vi "Draw All Bones.vi"(6 "Color":u32(colorbox)=16711680, 7 "Include Inferred Joints?":bool=TRUE, 8 "error in":errorcluster, 9 "Body Index":i32, 11 "Image":T1) -> (0 "error out":errorcluster, 3 "Image Out":T1)   [LabVIEW 2011, in "LVH-KinectOne.lvlib"]
uses:
  LVH-KinectOne.lvlib
  <vilib>/vision/Image Controls.llb/IMAQ Image.ctl
  Type Defs/JointType.ctl
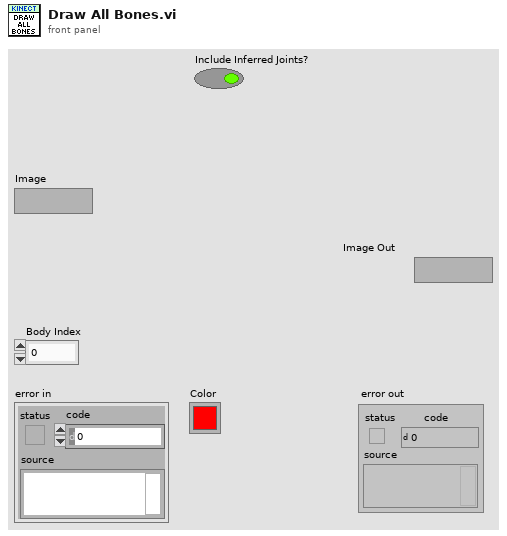
[diagram p1: front panel]
types:
  T1 = typedef "IMAQ Image.ctl" = refnum<image>
  T2 = typedef "LVH-KinectOne.lvlib/JointType.ctl" = i32
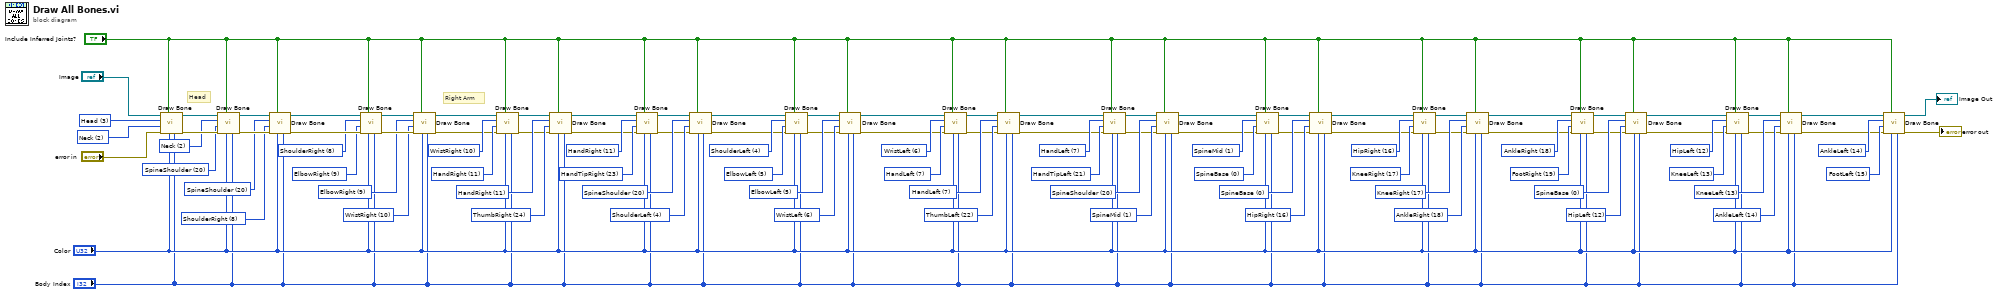
[diagram p0: block diagram]
diagram:
  w9 = T2 15 items=["SpineBase", "SpineMid", "Neck", "Head", "ShoulderLeft", "ElbowLeft", "WristLeft", "HandLeft", "ShoulderRight", "ElbowRight", "WristRight", "HandRight", "HipLeft", "KneeLeft", "AnkleLeft", "FootLeft", "HipRight", "KneeRight", "AnkleRight", "FootRight", "SpineShoulder", "HandTipLeft", "ThumbLeft", "HandTipRight", "ThumbRight"] ("Ending Joint")
  w8 = T2 14 items=["SpineBase", "SpineMid", "Neck", "Head", "ShoulderLeft", "ElbowLeft", "WristLeft", "HandLeft", "ShoulderRight", "ElbowRight", "WristRight", "HandRight", "HipLeft", "KneeLeft", "AnkleLeft", "FootLeft", "HipRight", "KneeRight", "AnkleRight", "FootRight", "SpineShoulder", "HandTipLeft", "ThumbLeft", "HandTipRight", "ThumbRight"] ("Starting Joint")
  w17 = T2 14 items=["SpineBase", "SpineMid", "Neck", "Head", "ShoulderLeft", "ElbowLeft", "WristLeft", "HandLeft", "ShoulderRight", "ElbowRight", "WristRight", "HandRight", "HipLeft", "KneeLeft", "AnkleLeft", "FootLeft", "HipRight", "KneeRight", "AnkleRight", "FootRight", "SpineShoulder", "HandTipLeft", "ThumbLeft", "HandTipRight", "ThumbRight"] ("Ending Joint")
  w16 = T2 13 items=["SpineBase", "SpineMid", "Neck", "Head", "ShoulderLeft", "ElbowLeft", "WristLeft", "HandLeft", "ShoulderRight", "ElbowRight", "WristRight", "HandRight", "HipLeft", "KneeLeft", "AnkleLeft", "FootLeft", "HipRight", "KneeRight", "AnkleRight", "FootRight", "SpineShoulder", "HandTipLeft", "ThumbLeft", "HandTipRight", "ThumbRight"] ("Starting Joint")
  w13 = T2 13 items=["SpineBase", "SpineMid", "Neck", "Head", "ShoulderLeft", "ElbowLeft", "WristLeft", "HandLeft", "ShoulderRight", "ElbowRight", "WristRight", "HandRight", "HipLeft", "KneeLeft", "AnkleLeft", "FootLeft", "HipRight", "KneeRight", "AnkleRight", "FootRight", "SpineShoulder", "HandTipLeft", "ThumbLeft", "HandTipRight", "ThumbRight"] ("Ending Joint")
  w12 = T2 12 items=["SpineBase", "SpineMid", "Neck", "Head", "ShoulderLeft", "ElbowLeft", "WristLeft", "HandLeft", "ShoulderRight", "ElbowRight", "WristRight", "HandRight", "HipLeft", "KneeLeft", "AnkleLeft", "FootLeft", "HipRight", "KneeRight", "AnkleRight", "FootRight", "SpineShoulder", "HandTipLeft", "ThumbLeft", "HandTipRight", "ThumbRight"] ("Starting Joint")
  w25 = T2 12 items=["SpineBase", "SpineMid", "Neck", "Head", "ShoulderLeft", "ElbowLeft", "WristLeft", "HandLeft", "ShoulderRight", "ElbowRight", "WristRight", "HandRight", "HipLeft", "KneeLeft", "AnkleLeft", "FootLeft", "HipRight", "KneeRight", "AnkleRight", "FootRight", "SpineShoulder", "HandTipLeft", "ThumbLeft", "HandTipRight", "ThumbRight"] ("Ending Joint")
  w24 = T2 0 items=["SpineBase", "SpineMid", "Neck", "Head", "ShoulderLeft", "ElbowLeft", "WristLeft", "HandLeft", "ShoulderRight", "ElbowRight", "WristRight", "HandRight", "HipLeft", "KneeLeft", "AnkleLeft", "FootLeft", "HipRight", "KneeRight", "AnkleRight", "FootRight", "SpineShoulder", "HandTipLeft", "ThumbLeft", "HandTipRight", "ThumbRight"] ("Starting Joint")
  w21 = T2 19 items=["SpineBase", "SpineMid", "Neck", "Head", "ShoulderLeft", "ElbowLeft", "WristLeft", "HandLeft", "ShoulderRight", "ElbowRight", "WristRight", "HandRight", "HipLeft", "KneeLeft", "AnkleLeft", "FootLeft", "HipRight", "KneeRight", "AnkleRight", "FootRight", "SpineShoulder", "HandTipLeft", "ThumbLeft", "HandTipRight", "ThumbRight"] ("Ending Joint")
  w20 = T2 18 items=["SpineBase", "SpineMid", "Neck", "Head", "ShoulderLeft", "ElbowLeft", "WristLeft", "HandLeft", "ShoulderRight", "ElbowRight", "WristRight", "HandRight", "HipLeft", "KneeLeft", "AnkleLeft", "FootLeft", "HipRight", "KneeRight", "AnkleRight", "FootRight", "SpineShoulder", "HandTipLeft", "ThumbLeft", "HandTipRight", "ThumbRight"] ("Starting Joint")
  w33 = T2 18 items=["SpineBase", "SpineMid", "Neck", "Head", "ShoulderLeft", "ElbowLeft", "WristLeft", "HandLeft", "ShoulderRight", "ElbowRight", "WristRight", "HandRight", "HipLeft", "KneeLeft", "AnkleLeft", "FootLeft", "HipRight", "KneeRight", "AnkleRight", "FootRight", "SpineShoulder", "HandTipLeft", "ThumbLeft", "HandTipRight", "ThumbRight"] ("Ending Joint")
  w32 = T2 17 items=["SpineBase", "SpineMid", "Neck", "Head", "ShoulderLeft", "ElbowLeft", "WristLeft", "HandLeft", "ShoulderRight", "ElbowRight", "WristRight", "HandRight", "HipLeft", "KneeLeft", "AnkleLeft", "FootLeft", "HipRight", "KneeRight", "AnkleRight", "FootRight", "SpineShoulder", "HandTipLeft", "ThumbLeft", "HandTipRight", "ThumbRight"] ("Starting Joint")
  w29 = T2 17 items=["SpineBase", "SpineMid", "Neck", "Head", "ShoulderLeft", "ElbowLeft", "WristLeft", "HandLeft", "ShoulderRight", "ElbowRight", "WristRight", "HandRight", "HipLeft", "KneeLeft", "AnkleLeft", "FootLeft", "HipRight", "KneeRight", "AnkleRight", "FootRight", "SpineShoulder", "HandTipLeft", "ThumbLeft", "HandTipRight", "ThumbRight"] ("Ending Joint")
  w28 = T2 16 items=["SpineBase", "SpineMid", "Neck", "Head", "ShoulderLeft", "ElbowLeft", "WristLeft", "HandLeft", "ShoulderRight", "ElbowRight", "WristRight", "HandRight", "HipLeft", "KneeLeft", "AnkleLeft", "FootLeft", "HipRight", "KneeRight", "AnkleRight", "FootRight", "SpineShoulder", "HandTipLeft", "ThumbLeft", "HandTipRight", "ThumbRight"] ("Starting Joint")
  w41 = T2 16 items=["SpineBase", "SpineMid", "Neck", "Head", "ShoulderLeft", "ElbowLeft", "WristLeft", "HandLeft", "ShoulderRight", "ElbowRight", "WristRight", "HandRight", "HipLeft", "KneeLeft", "AnkleLeft", "FootLeft", "HipRight", "KneeRight", "AnkleRight", "FootRight", "SpineShoulder", "HandTipLeft", "ThumbLeft", "HandTipRight", "ThumbRight"] ("Ending Joint")
  w40 = T2 0 items=["SpineBase", "SpineMid", "Neck", "Head", "ShoulderLeft", "ElbowLeft", "WristLeft", "HandLeft", "ShoulderRight", "ElbowRight", "WristRight", "HandRight", "HipLeft", "KneeLeft", "AnkleLeft", "FootLeft", "HipRight", "KneeRight", "AnkleRight", "FootRight", "SpineShoulder", "HandTipLeft", "ThumbLeft", "HandTipRight", "ThumbRight"] ("Starting Joint")
  w37 = T2 0 items=["SpineBase", "SpineMid", "Neck", "Head", "ShoulderLeft", "ElbowLeft", "WristLeft", "HandLeft", "ShoulderRight", "ElbowRight", "WristRight", "HandRight", "HipLeft", "KneeLeft", "AnkleLeft", "FootLeft", "HipRight", "KneeRight", "AnkleRight", "FootRight", "SpineShoulder", "HandTipLeft", "ThumbLeft", "HandTipRight", "ThumbRight"] ("Ending Joint")
  w36 = T2 1 items=["SpineBase", "SpineMid", "Neck", "Head", "ShoulderLeft", "ElbowLeft", "WristLeft", "HandLeft", "ShoulderRight", "ElbowRight", "WristRight", "HandRight", "HipLeft", "KneeLeft", "AnkleLeft", "FootLeft", "HipRight", "KneeRight", "AnkleRight", "FootRight", "SpineShoulder", "HandTipLeft", "ThumbLeft", "HandTipRight", "ThumbRight"] ("Starting Joint")
  w49 = T2 1 items=["SpineBase", "SpineMid", "Neck", "Head", "ShoulderLeft", "ElbowLeft", "WristLeft", "HandLeft", "ShoulderRight", "ElbowRight", "WristRight", "HandRight", "HipLeft", "KneeLeft", "AnkleLeft", "FootLeft", "HipRight", "KneeRight", "AnkleRight", "FootRight", "SpineShoulder", "HandTipLeft", "ThumbLeft", "HandTipRight", "ThumbRight"] ("Ending Joint")
  w48 = T2 20 items=["SpineBase", "SpineMid", "Neck", "Head", "ShoulderLeft", "ElbowLeft", "WristLeft", "HandLeft", "ShoulderRight", "ElbowRight", "WristRight", "HandRight", "HipLeft", "KneeLeft", "AnkleLeft", "FootLeft", "HipRight", "KneeRight", "AnkleRight", "FootRight", "SpineShoulder", "HandTipLeft", "ThumbLeft", "HandTipRight", "ThumbRight"] ("Starting Joint")
  w45 = T2 21 items=["SpineBase", "SpineMid", "Neck", "Head", "ShoulderLeft", "ElbowLeft", "WristLeft", "HandLeft", "ShoulderRight", "ElbowRight", "WristRight", "HandRight", "HipLeft", "KneeLeft", "AnkleLeft", "FootLeft", "HipRight", "KneeRight", "AnkleRight", "FootRight", "SpineShoulder", "HandTipLeft", "ThumbLeft", "HandTipRight", "ThumbRight"] ("Ending Joint")
  w44 = T2 7 items=["SpineBase", "SpineMid", "Neck", "Head", "ShoulderLeft", "ElbowLeft", "WristLeft", "HandLeft", "ShoulderRight", "ElbowRight", "WristRight", "HandRight", "HipLeft", "KneeLeft", "AnkleLeft", "FootLeft", "HipRight", "KneeRight", "AnkleRight", "FootRight", "SpineShoulder", "HandTipLeft", "ThumbLeft", "HandTipRight", "ThumbRight"] ("Starting Joint")
  w57 = T2 22 items=["SpineBase", "SpineMid", "Neck", "Head", "ShoulderLeft", "ElbowLeft", "WristLeft", "HandLeft", "ShoulderRight", "ElbowRight", "WristRight", "HandRight", "HipLeft", "KneeLeft", "AnkleLeft", "FootLeft", "HipRight", "KneeRight", "AnkleRight", "FootRight", "SpineShoulder", "HandTipLeft", "ThumbLeft", "HandTipRight", "ThumbRight"] ("Ending Joint")
  w56 = T2 7 items=["SpineBase", "SpineMid", "Neck", "Head", "ShoulderLeft", "ElbowLeft", "WristLeft", "HandLeft", "ShoulderRight", "ElbowRight", "WristRight", "HandRight", "HipLeft", "KneeLeft", "AnkleLeft", "FootLeft", "HipRight", "KneeRight", "AnkleRight", "FootRight", "SpineShoulder", "HandTipLeft", "ThumbLeft", "HandTipRight", "ThumbRight"] ("Starting Joint")
  w53 = T2 7 items=["SpineBase", "SpineMid", "Neck", "Head", "ShoulderLeft", "ElbowLeft", "WristLeft", "HandLeft", "ShoulderRight", "ElbowRight", "WristRight", "HandRight", "HipLeft", "KneeLeft", "AnkleLeft", "FootLeft", "HipRight", "KneeRight", "AnkleRight", "FootRight", "SpineShoulder", "HandTipLeft", "ThumbLeft", "HandTipRight", "ThumbRight"] ("Ending Joint")
  w52 = T2 6 items=["SpineBase", "SpineMid", "Neck", "Head", "ShoulderLeft", "ElbowLeft", "WristLeft", "HandLeft", "ShoulderRight", "ElbowRight", "WristRight", "HandRight", "HipLeft", "KneeLeft", "AnkleLeft", "FootLeft", "HipRight", "KneeRight", "AnkleRight", "FootRight", "SpineShoulder", "HandTipLeft", "ThumbLeft", "HandTipRight", "ThumbRight"] ("Starting Joint")
  w65 = T2 6 items=["SpineBase", "SpineMid", "Neck", "Head", "ShoulderLeft", "ElbowLeft", "WristLeft", "HandLeft", "ShoulderRight", "ElbowRight", "WristRight", "HandRight", "HipLeft", "KneeLeft", "AnkleLeft", "FootLeft", "HipRight", "KneeRight", "AnkleRight", "FootRight", "SpineShoulder", "HandTipLeft", "ThumbLeft", "HandTipRight", "ThumbRight"] ("Ending Joint")
  w64 = T2 5 items=["SpineBase", "SpineMid", "Neck", "Head", "ShoulderLeft", "ElbowLeft", "WristLeft", "HandLeft", "ShoulderRight", "ElbowRight", "WristRight", "HandRight", "HipLeft", "KneeLeft", "AnkleLeft", "FootLeft", "HipRight", "KneeRight", "AnkleRight", "FootRight", "SpineShoulder", "HandTipLeft", "ThumbLeft", "HandTipRight", "ThumbRight"] ("Starting Joint")
  w61 = T2 5 items=["SpineBase", "SpineMid", "Neck", "Head", "ShoulderLeft", "ElbowLeft", "WristLeft", "HandLeft", "ShoulderRight", "ElbowRight", "WristRight", "HandRight", "HipLeft", "KneeLeft", "AnkleLeft", "FootLeft", "HipRight", "KneeRight", "AnkleRight", "FootRight", "SpineShoulder", "HandTipLeft", "ThumbLeft", "HandTipRight", "ThumbRight"] ("Ending Joint")
  w60 = T2 4 items=["SpineBase", "SpineMid", "Neck", "Head", "ShoulderLeft", "ElbowLeft", "WristLeft", "HandLeft", "ShoulderRight", "ElbowRight", "WristRight", "HandRight", "HipLeft", "KneeLeft", "AnkleLeft", "FootLeft", "HipRight", "KneeRight", "AnkleRight", "FootRight", "SpineShoulder", "HandTipLeft", "ThumbLeft", "HandTipRight", "ThumbRight"] ("Starting Joint")
  w74 = T2 4 items=["SpineBase", "SpineMid", "Neck", "Head", "ShoulderLeft", "ElbowLeft", "WristLeft", "HandLeft", "ShoulderRight", "ElbowRight", "WristRight", "HandRight", "HipLeft", "KneeLeft", "AnkleLeft", "FootLeft", "HipRight", "KneeRight", "AnkleRight", "FootRight", "SpineShoulder", "HandTipLeft", "ThumbLeft", "HandTipRight", "ThumbRight"] ("Ending Joint")
  w73 = T2 20 items=["SpineBase", "SpineMid", "Neck", "Head", "ShoulderLeft", "ElbowLeft", "WristLeft", "HandLeft", "ShoulderRight", "ElbowRight", "WristRight", "HandRight", "HipLeft", "KneeLeft", "AnkleLeft", "FootLeft", "HipRight", "KneeRight", "AnkleRight", "FootRight", "SpineShoulder", "HandTipLeft", "ThumbLeft", "HandTipRight", "ThumbRight"] ("Starting Joint")
  w70 = T2 23 items=["SpineBase", "SpineMid", "Neck", "Head", "ShoulderLeft", "ElbowLeft", "WristLeft", "HandLeft", "ShoulderRight", "ElbowRight", "WristRight", "HandRight", "HipLeft", "KneeLeft", "AnkleLeft", "FootLeft", "HipRight", "KneeRight", "AnkleRight", "FootRight", "SpineShoulder", "HandTipLeft", "ThumbLeft", "HandTipRight", "ThumbRight"] ("Ending Joint")
  w69 = T2 11 items=["SpineBase", "SpineMid", "Neck", "Head", "ShoulderLeft", "ElbowLeft", "WristLeft", "HandLeft", "ShoulderRight", "ElbowRight", "WristRight", "HandRight", "HipLeft", "KneeLeft", "AnkleLeft", "FootLeft", "HipRight", "KneeRight", "AnkleRight", "FootRight", "SpineShoulder", "HandTipLeft", "ThumbLeft", "HandTipRight", "ThumbRight"] ("Starting Joint")
  w81 = T2 24 items=["SpineBase", "SpineMid", "Neck", "Head", "ShoulderLeft", "ElbowLeft", "WristLeft", "HandLeft", "ShoulderRight", "ElbowRight", "WristRight", "HandRight", "HipLeft", "KneeLeft", "AnkleLeft", "FootLeft", "HipRight", "KneeRight", "AnkleRight", "FootRight", "SpineShoulder", "HandTipLeft", "ThumbLeft", "HandTipRight", "ThumbRight"] ("Ending Joint")
  w80 = T2 11 items=["SpineBase", "SpineMid", "Neck", "Head", "ShoulderLeft", "ElbowLeft", "WristLeft", "HandLeft", "ShoulderRight", "ElbowRight", "WristRight", "HandRight", "HipLeft", "KneeLeft", "AnkleLeft", "FootLeft", "HipRight", "KneeRight", "AnkleRight", "FootRight", "SpineShoulder", "HandTipLeft", "ThumbLeft", "HandTipRight", "ThumbRight"] ("Starting Joint")
  w77 = T2 11 items=["SpineBase", "SpineMid", "Neck", "Head", "ShoulderLeft", "ElbowLeft", "WristLeft", "HandLeft", "ShoulderRight", "ElbowRight", "WristRight", "HandRight", "HipLeft", "KneeLeft", "AnkleLeft", "FootLeft", "HipRight", "KneeRight", "AnkleRight", "FootRight", "SpineShoulder", "HandTipLeft", "ThumbLeft", "HandTipRight", "ThumbRight"] ("Ending Joint")
  w76 = T2 10 items=["SpineBase", "SpineMid", "Neck", "Head", "ShoulderLeft", "ElbowLeft", "WristLeft", "HandLeft", "ShoulderRight", "ElbowRight", "WristRight", "HandRight", "HipLeft", "KneeLeft", "AnkleLeft", "FootLeft", "HipRight", "KneeRight", "AnkleRight", "FootRight", "SpineShoulder", "HandTipLeft", "ThumbLeft", "HandTipRight", "ThumbRight"] ("Starting Joint")
  w82 = T2 10 items=["SpineBase", "SpineMid", "Neck", "Head", "ShoulderLeft", "ElbowLeft", "WristLeft", "HandLeft", "ShoulderRight", "ElbowRight", "WristRight", "HandRight", "HipLeft", "KneeLeft", "AnkleLeft", "FootLeft", "HipRight", "KneeRight", "AnkleRight", "FootRight", "SpineShoulder", "HandTipLeft", "ThumbLeft", "HandTipRight", "ThumbRight"] ("Ending Joint")
  w83 = T2 9 items=["SpineBase", "SpineMid", "Neck", "Head", "ShoulderLeft", "ElbowLeft", "WristLeft", "HandLeft", "ShoulderRight", "ElbowRight", "WristRight", "HandRight", "HipLeft", "KneeLeft", "AnkleLeft", "FootLeft", "HipRight", "KneeRight", "AnkleRight", "FootRight", "SpineShoulder", "HandTipLeft", "ThumbLeft", "HandTipRight", "ThumbRight"] ("JointType")
  w86 = T2 9 items=["SpineBase", "SpineMid", "Neck", "Head", "ShoulderLeft", "ElbowLeft", "WristLeft", "HandLeft", "ShoulderRight", "ElbowRight", "WristRight", "HandRight", "HipLeft", "KneeLeft", "AnkleLeft", "FootLeft", "HipRight", "KneeRight", "AnkleRight", "FootRight", "SpineShoulder", "HandTipLeft", "ThumbLeft", "HandTipRight", "ThumbRight"] ("Ending Joint")
  w87 = T2 8 items=["SpineBase", "SpineMid", "Neck", "Head", "ShoulderLeft", "ElbowLeft", "WristLeft", "HandLeft", "ShoulderRight", "ElbowRight", "WristRight", "HandRight", "HipLeft", "KneeLeft", "AnkleLeft", "FootLeft", "HipRight", "KneeRight", "AnkleRight", "FootRight", "SpineShoulder", "HandTipLeft", "ThumbLeft", "HandTipRight", "ThumbRight"] ("JointType")
  w90 = T2 8 items=["SpineBase", "SpineMid", "Neck", "Head", "ShoulderLeft", "ElbowLeft", "WristLeft", "HandLeft", "ShoulderRight", "ElbowRight", "WristRight", "HandRight", "HipLeft", "KneeLeft", "AnkleLeft", "FootLeft", "HipRight", "KneeRight", "AnkleRight", "FootRight", "SpineShoulder", "HandTipLeft", "ThumbLeft", "HandTipRight", "ThumbRight"] ("Ending Joint")
  w91 = T2 20 items=["SpineBase", "SpineMid", "Neck", "Head", "ShoulderLeft", "ElbowLeft", "WristLeft", "HandLeft", "ShoulderRight", "ElbowRight", "WristRight", "HandRight", "HipLeft", "KneeLeft", "AnkleLeft", "FootLeft", "HipRight", "KneeRight", "AnkleRight", "FootRight", "SpineShoulder", "HandTipLeft", "ThumbLeft", "HandTipRight", "ThumbRight"] ("JointType")
  w94 = T2 20 items=["SpineBase", "SpineMid", "Neck", "Head", "ShoulderLeft", "ElbowLeft", "WristLeft", "HandLeft", "ShoulderRight", "ElbowRight", "WristRight", "HandRight", "HipLeft", "KneeLeft", "AnkleLeft", "FootLeft", "HipRight", "KneeRight", "AnkleRight", "FootRight", "SpineShoulder", "HandTipLeft", "ThumbLeft", "HandTipRight", "ThumbRight"] ("Ending Joint")
  w95 = T2 2 items=["SpineBase", "SpineMid", "Neck", "Head", "ShoulderLeft", "ElbowLeft", "WristLeft", "HandLeft", "ShoulderRight", "ElbowRight", "WristRight", "HandRight", "HipLeft", "KneeLeft", "AnkleLeft", "FootLeft", "HipRight", "KneeRight", "AnkleRight", "FootRight", "SpineShoulder", "HandTipLeft", "ThumbLeft", "HandTipRight", "ThumbRight"] ("JointType")
  w99 = T2 2 items=["SpineBase", "SpineMid", "Neck", "Head", "ShoulderLeft", "ElbowLeft", "WristLeft", "HandLeft", "ShoulderRight", "ElbowRight", "WristRight", "HandRight", "HipLeft", "KneeLeft", "AnkleLeft", "FootLeft", "HipRight", "KneeRight", "AnkleRight", "FootRight", "SpineShoulder", "HandTipLeft", "ThumbLeft", "HandTipRight", "ThumbRight"] ("Ending Joint")
  w100 = T2 3 items=["SpineBase", "SpineMid", "Neck", "Head", "ShoulderLeft", "ElbowLeft", "WristLeft", "HandLeft", "ShoulderRight", "ElbowRight", "WristRight", "HandRight", "HipLeft", "KneeLeft", "AnkleLeft", "FootLeft", "HipRight", "KneeRight", "AnkleRight", "FootRight", "SpineShoulder", "HandTipLeft", "ThumbLeft", "HandTipRight", "ThumbRight"] ("JointType")
  # "Right Arm"
  # "Head"
  n1 = call "Draw Bone.vi"("Body Index"="Body Index", "Color"="Color", "Include Inferred Joints?"="Include Inferred Joints?", "error in"="error in", "Ending Joint"=w99, "Starting Joint"=w100, "Image"="Image") -> ("error out"=w97:errorcluster, "Image Out"=w96:T1)  [unwired: 3 in]
  n2 = call "Draw Bone.vi"("Body Index"="Body Index", "Color"="Color", "Include Inferred Joints?"="Include Inferred Joints?", "error in"=w97, "Ending Joint"=w94, "Starting Joint"=w95, "Image"=w96) -> ("error out"=w93:errorcluster, "Image Out"=w92:T1)  [unwired: 3 in]
  n3 = call "Draw Bone.vi"("Body Index"="Body Index", "Color"="Color", "Include Inferred Joints?"="Include Inferred Joints?", "error in"=w93, "Ending Joint"=w90, "Starting Joint"=w91, "Image"=w92) -> ("error out"=w89:errorcluster, "Image Out"=w88:T1)  [unwired: 3 in]
  n4 = call "Draw Bone.vi"("Body Index"="Body Index", "Color"="Color", "Include Inferred Joints?"="Include Inferred Joints?", "error in"=w89, "Ending Joint"=w86, "Starting Joint"=w87, "Image"=w88) -> ("error out"=w85:errorcluster, "Image Out"=w84:T1)  [unwired: 3 in]
  n5 = call "Draw Bone.vi"("Body Index"="Body Index", "Color"="Color", "Include Inferred Joints?"="Include Inferred Joints?", "error in"=w85, "Ending Joint"=w82, "Starting Joint"=w83, "Image"=w84) -> ("error out"=w75:errorcluster, "Image Out"=w67:T1)  [unwired: 3 in]
  n6 = call "Draw Bone.vi"("Body Index"="Body Index", "Color"="Color", "Include Inferred Joints?"="Include Inferred Joints?", "error in"=w75, "Ending Joint"=w77, "Starting Joint"=w76, "Image"=w67) -> ("error out"=w78:errorcluster, "Image Out"=w79:T1)  [unwired: 3 in]
  n7 = call "Draw Bone.vi"("Body Index"="Body Index", "Color"="Color", "Include Inferred Joints?"="Include Inferred Joints?", "error in"=w78, "Ending Joint"=w81, "Starting Joint"=w80, "Image"=w79) -> ("error out"=w68:errorcluster, "Image Out"=w66:T1)  [unwired: 3 in]
  n8 = call "Draw Bone.vi"("Body Index"="Body Index", "Color"="Color", "Include Inferred Joints?"="Include Inferred Joints?", "error in"=w68, "Ending Joint"=w70, "Starting Joint"=w69, "Image"=w66) -> ("error out"=w71:errorcluster, "Image Out"=w72:T1)  [unwired: 3 in]
  n9 = call "Draw Bone.vi"("Body Index"="Body Index", "Color"="Color", "Include Inferred Joints?"="Include Inferred Joints?", "error in"=w71, "Ending Joint"=w74, "Starting Joint"=w73, "Image"=w72) -> ("error out"=w59:errorcluster, "Image Out"=w58:T1)  [unwired: 3 in]
  n10 = call "Draw Bone.vi"("Body Index"="Body Index", "Color"="Color", "Include Inferred Joints?"="Include Inferred Joints?", "error in"=w59, "Ending Joint"=w61, "Starting Joint"=w60, "Image"=w58) -> ("error out"=w62:errorcluster, "Image Out"=w63:T1)  [unwired: 3 in]
  n11 = call "Draw Bone.vi"("Body Index"="Body Index", "Color"="Color", "Include Inferred Joints?"="Include Inferred Joints?", "error in"=w62, "Ending Joint"=w65, "Starting Joint"=w64, "Image"=w63) -> ("error out"=w51:errorcluster, "Image Out"=w50:T1)  [unwired: 3 in]
  n12 = call "Draw Bone.vi"("Body Index"="Body Index", "Color"="Color", "Include Inferred Joints?"="Include Inferred Joints?", "error in"=w51, "Ending Joint"=w53, "Starting Joint"=w52, "Image"=w50) -> ("error out"=w54:errorcluster, "Image Out"=w55:T1)  [unwired: 3 in]
  n13 = call "Draw Bone.vi"("Body Index"="Body Index", "Color"="Color", "Include Inferred Joints?"="Include Inferred Joints?", "error in"=w54, "Ending Joint"=w57, "Starting Joint"=w56, "Image"=w55) -> ("error out"=w43:errorcluster, "Image Out"=w42:T1)  [unwired: 3 in]
  n14 = call "Draw Bone.vi"("Body Index"="Body Index", "Color"="Color", "Include Inferred Joints?"="Include Inferred Joints?", "error in"=w43, "Ending Joint"=w45, "Starting Joint"=w44, "Image"=w42) -> ("error out"=w46:errorcluster, "Image Out"=w47:T1)  [unwired: 3 in]
  n15 = call "Draw Bone.vi"("Body Index"="Body Index", "Color"="Color", "Include Inferred Joints?"="Include Inferred Joints?", "error in"=w46, "Ending Joint"=w49, "Starting Joint"=w48, "Image"=w47) -> ("error out"=w34:errorcluster, "Image Out"=w35:T1)  [unwired: 3 in]
  n16 = call "Draw Bone.vi"("Body Index"="Body Index", "Color"="Color", "Include Inferred Joints?"="Include Inferred Joints?", "error in"=w34, "Ending Joint"=w37, "Starting Joint"=w36, "Image"=w35) -> ("error out"=w38:errorcluster, "Image Out"=w39:T1)  [unwired: 3 in]
  n17 = call "Draw Bone.vi"("Body Index"="Body Index", "Color"="Color", "Include Inferred Joints?"="Include Inferred Joints?", "error in"=w38, "Ending Joint"=w41, "Starting Joint"=w40, "Image"=w39) -> ("error out"=w27:errorcluster, "Image Out"=w26:T1)  [unwired: 3 in]
  n18 = call "Draw Bone.vi"("Body Index"="Body Index", "Color"="Color", "Include Inferred Joints?"="Include Inferred Joints?", "error in"=w27, "Ending Joint"=w29, "Starting Joint"=w28, "Image"=w26) -> ("error out"=w30:errorcluster, "Image Out"=w31:T1)  [unwired: 3 in]
  n19 = call "Draw Bone.vi"("Body Index"="Body Index", "Color"="Color", "Include Inferred Joints?"="Include Inferred Joints?", "error in"=w30, "Ending Joint"=w33, "Starting Joint"=w32, "Image"=w31) -> ("error out"=w19:errorcluster, "Image Out"=w18:T1)  [unwired: 3 in]
  n20 = call "Draw Bone.vi"("Body Index"="Body Index", "Color"="Color", "Include Inferred Joints?"="Include Inferred Joints?", "error in"=w19, "Ending Joint"=w21, "Starting Joint"=w20, "Image"=w18) -> ("error out"=w22:errorcluster, "Image Out"=w23:T1)  [unwired: 3 in]
  n21 = call "Draw Bone.vi"("Body Index"="Body Index", "Color"="Color", "Include Inferred Joints?"="Include Inferred Joints?", "error in"=w22, "Ending Joint"=w25, "Starting Joint"=w24, "Image"=w23) -> ("error out"=w10:errorcluster, "Image Out"=w11:T1)  [unwired: 3 in]
  n22 = call "Draw Bone.vi"("Body Index"="Body Index", "Color"="Color", "Include Inferred Joints?"="Include Inferred Joints?", "error in"=w10, "Ending Joint"=w13, "Starting Joint"=w12, "Image"=w11) -> ("error out"=w14:errorcluster, "Image Out"=w15:T1)  [unwired: 3 in]
  n23 = call "Draw Bone.vi"("Body Index"="Body Index", "Color"="Color", "Include Inferred Joints?"="Include Inferred Joints?", "error in"=w14, "Ending Joint"=w17, "Starting Joint"=w16, "Image"=w15) -> ("error out"=w7:errorcluster, "Image Out"=w6:T1)  [unwired: 3 in]
  n24 = call "Draw Bone.vi"("Body Index"="Body Index", "Color"="Color", "Include Inferred Joints?"="Include Inferred Joints?", "error in"=w7, "Ending Joint"=w9, "Starting Joint"=w8, "Image"=w6) -> ("error out"=→"error out":errorcluster, "Image Out"=→"Image Out":T1)  [unwired: 3 in]
